vi "Check Still Available.vi"(8 "error in (no error)":errorcluster, 11 "test_hardwareactor in":refnum<class "test_hardwareactor.lvclass">) -> (0 "error out":errorcluster, 3 "test_hardwareactor out":refnum<class "test_hardwareactor.lvclass">)   [LabVIEW 2015, in "test_hardwareactor.lvclass"]
uses:
  test_hardwareactor.lvclass
  Output Actor Hardware/Output Actor Hardware.lvclass
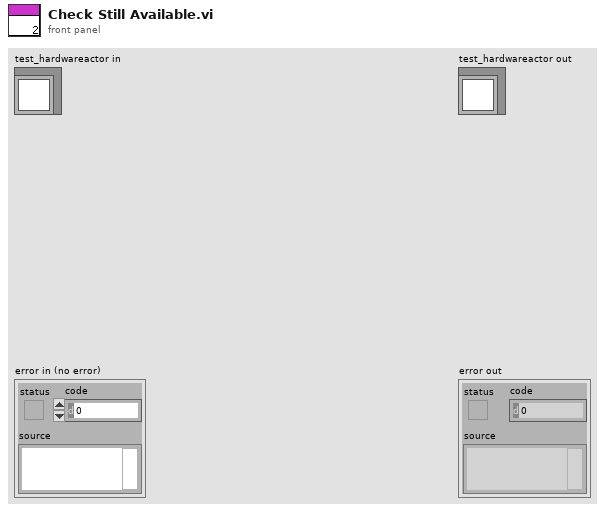
[diagram p1: front panel]
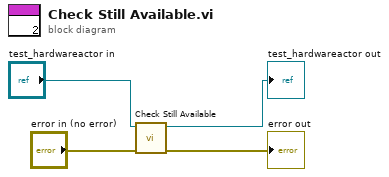
[diagram p0: block diagram]
diagram:
  n1 = call-parent "Check Still Available.vi"("error in (no error)"="error in (no error)", "Output Actor Hardware in"="test_hardwareactor in") -> ("error out"=→"error out":errorcluster, "Output Actor Hardware out"=→"test_hardwareactor out":refnum<class "test_hardwareactor.lvclass">)  [unwired: 8 in]
